vi "Initialize with Switch Parameters.vi"(8 "error in (no error)":errorcluster, 10 "Switch Parameters in":refnum<class "Abstract Switch Init Parameters.lvclass">, 11 "Abstract Switch Consumer in":refnum<class "Abstract Switch Consumer.lvclass">) -> (0 "error out":errorcluster, 3 "Abstract Switch Consumer out":refnum<class "Abstract Switch Consumer.lvclass">)   [LabVIEW 2017, in "Messaging.lvlib" / "Abstract Switch Consumer.lvclass"]
uses:
  Abstract Switch Consumer.lvclass
  Abstract Switch Init Parameters/Abstract Switch Init Parameters.lvclass
  Abstract Switch Consumer.lvclass/Abstract Switch Consumer.ctl
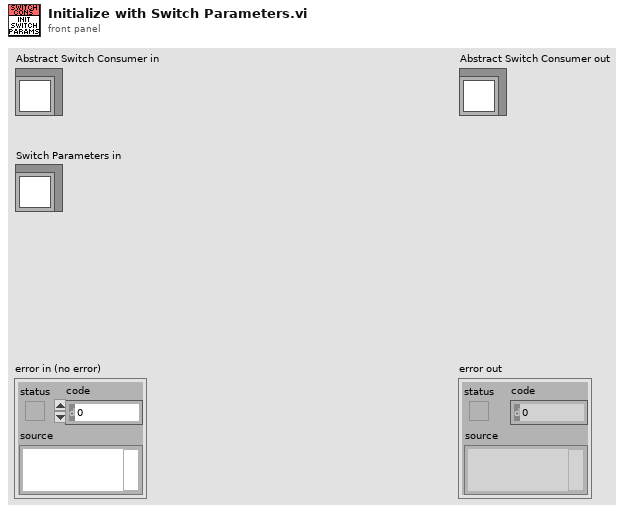
[diagram p1: front panel]
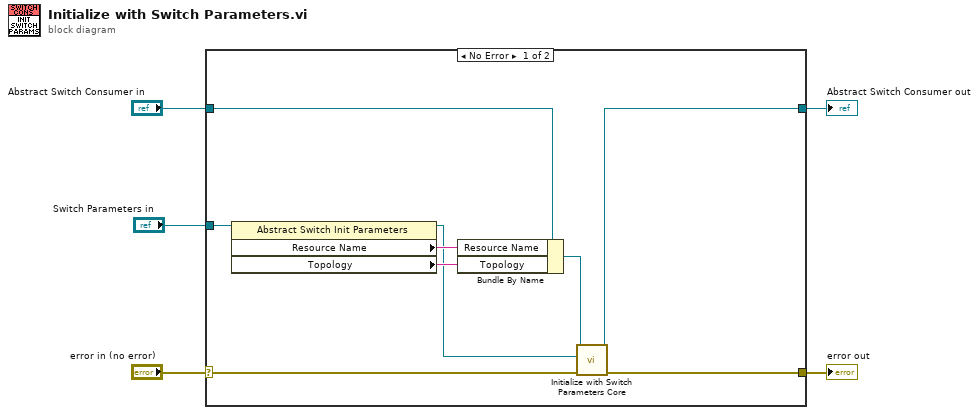
[diagram p0: block diagram]
diagram:
  n1 = case shown="No Error" "error in (no error)" {
    selector: "error in (no error)" -> [w6 w16]
    tunnel: [w10 w16] -> w4
    tunnel: [w8 w15] -> w2
    tunnel: "Abstract Switch Consumer in" -> [w13 w15]
    tunnel: "Switch Parameters in" -> [w14 _]
    frame No Error {
      n2 = property class="Abstract Switch Init Parameters"(reference=w14) -> (reference out=w7:refnum<class "Abstract Switch Init Parameters.lvclass">, "Resource Name"=w12:string, "Topology"=w11:string)  [unwired: 1 in, 1 out]
      n3 = Bundle By Name(cluster=w13, "Resource Name"=w12, "Topology"=w11) -> (w9:refnum<class "Abstract Switch Consumer.lvclass">)
      n4 = call-dynamic "Initialize with Switch Parameters Core.vi"("error in (no error)"=w6, "Switch Parameters in"=w7, "Abstract Switch Consumer in"=w9) -> ("error out"=w10:errorcluster, "Abstract Switch Consumer out"=w8:refnum<class "Abstract Switch Consumer.lvclass">)  [unwired: 7 in]
    }
    frame Error {
    }
  }
  "error out" <- w4
  "Abstract Switch Consumer out" <- w2
